vi "FRCts20_Backend_RequestRoot_GET.vi"(6 "Message Attributes":T4, 8 "error in (no error)":errorcluster, 10 "Data":string, 11 "Engine_Refnums":T1) -> (0 "error out":errorcluster)   [LabVIEW 2013, in "FRCts20_Backend_Engine.lvlib"]
doc: "Returns all requests' data, called by the Request Root API. Expects no inputs"
uses:
  FRCts20_Backend_Engine.lvlib
  Dependencies/Keyed Array/KeyedArray.ctl
  FRCts20_Backend_EngineRefnums.ctl
  INI_Accessor/FRCts20_Backend_INI Controller.lvclass
  Dependencies/AMC/_SubVIs/TypeDefs/Message Queue.ctl
  Dependencies/AMC/_SubVIs/TypeDefs/Message.ctl
  <vilib>/addons/database/Connection.llb/Conn ObjectReference.ctl
  FRCts20_Backend_FGVOperation.ctl
  FRCts20_Backend_API/FRCts20_Backend_API_RequestRoot.ctl
  FRCts20_Backend_API/FRCts20_Backend_API_Status.ctl
  FRCts20_Backend_API/FRCts20_Backend_API.lvlib
  Dependencies/Keyed Array/Tools_KeyedArray.lvlib
  Dependencies/AMC/AMC.lvlib
  <vilib>/addons/database/NI_Database_API.lvlib
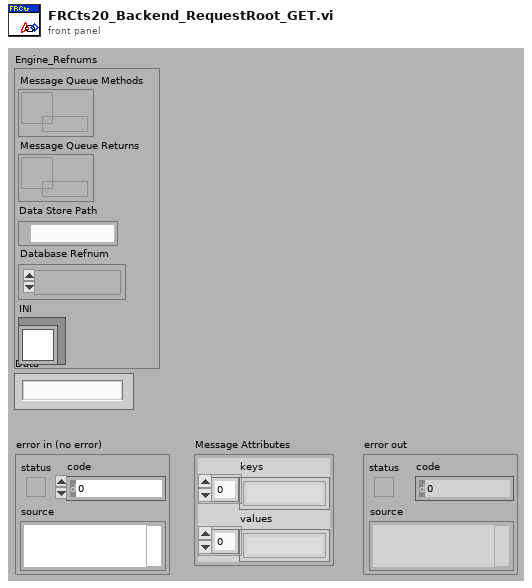
[diagram p1: front panel]
types:
  T1 = typedef "FRCts20_Backend_Engine.lvlib/FRCts20_Backend_EngineRefnums.ctl" = cluster{"Message Queue Methods":T2, "Message Queue Returns":T2, "Data Store Path":path, "Database Refnum":T3, "INI":refnum<class "FRCts20_Backend_INI Controller.lvclass">}
  T2 = typedef "AMC.lvlib/Message Queue.ctl" = refnum<queue>
  T3 = typedef "NI_Database_API.lvlib/Conn ObjectReference.ctl" = refnum<k1>
  T4 = typedef "Tools_KeyedArray.lvlib/KeyedArray.ctl" = cluster{"keys":string[], "values":string[]}
  T5 = typedef "FRCts20_Backend_Engine.lvlib/FRCts20_Backend_FGVOperation.ctl" = enum16{"Initialize", "EnqueueMessage", "EnqueueDataReturn", "FlushMessage", "FlushDataReturn"}
  T6 = typedef "FRCts20_Backend_API.lvlib/FRCts20_Backend_API_RequestRoot.ctl" = cluster{"Requests":cluster{"Request Index":u32, "Description":string, "Status":T7, "Open Date":timestamp, "Last Update":timestamp, "Closed Date":timestamp, "Team Index":u32}[], "APIReturn":string}
  T7 = typedef "FRCts20_Backend_API.lvlib/FRCts20_Backend_API_Status.ctl" = enum16{"Open", "In Work", "Closed"}
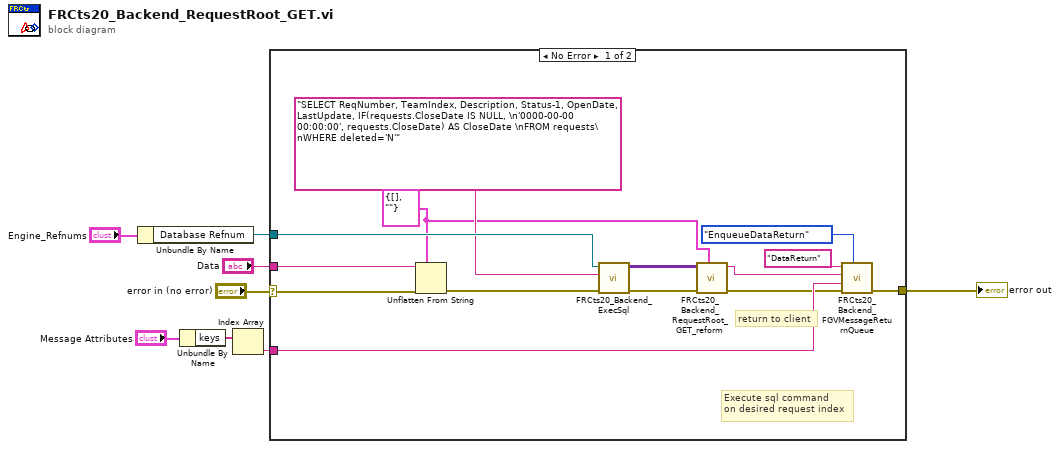
[diagram p0: block diagram]
diagram:
  n1 = Unbundle By Name("Engine_Refnums") -> ("Database Refnum"=w1:T3)
  n2 = Unbundle By Name("Message Attributes") -> ("keys"=w4:string[])
  n3 = Index Array(array=w4) -> (element=w3:string)  [unwired: 1 in]
  n4 = case shown="No Error" "error in (no error)" {
    selector: "error in (no error)" -> [w19 w23]
    tunnel: [w22 w23] -> w7
    tunnel: w1 -> [w14 _]
    tunnel: "Data" -> [w20 _]
    tunnel: w3 -> [w21 _]
    frame No Error {
      w9 = T6 {"Requests"=[], "APIReturn"=""} ("Request Root")
      # "return to client"
      # "Execute sql command\non desired request index"
      n5 = Unflatten From String(type=w9, binary string=w20, error in (no error)=w19) -> (error out=w10:errorcluster)  [unwired: 2 in, 2 out]
      n6 = call "FRCts20_Backend_ExecSql.vi"("error in (no error)"=w10, "format string"="SELECT ReqNumber, TeamIndex, Description, Status-1, OpenDate, LastUpdate, IF(requests.CloseDate IS NULL, \n'0000-00-00 00:00:00', requests.CloseDate) AS CloseDate \nFROM requests\nWHERE deleted='N'", "Refnum in"=w14) -> ("error out"=w12:errorcluster, "recordset data"=w13:variant[][])  [unwired: 6 in, 1 out]
      n7 = call "FRCts20_Backend_RequestRoot_GET_reform.vi"("Request Root"=w9, "error in (no error)"=w12, "recordset data"=w13) -> ("error out"=w15:errorcluster, "data string"=w16:string)  [unwired: 7 in]
      n8 = call "FRCts20_Backend_FGVMessageReturnQueue.vi"("Operation"=FRCts20_Backend_FGVOperation."EnqueueDataReturn", "error in (no error)"=w15, "Key"=w21, "Message Value"=w16, "Message Name"="DataReturn") -> ("error out"=w22:errorcluster)  [unwired: 5 in, 1 out]
    }
    frame Error {
    }
  }
  "error out" <- w7
